vi "Enqueue Message.vi"   [LabVIEW 2024, in "AA PM Message Queue.lvlib"]
doc: "For a regular message, enqueue the message. For a priority message, enqueue it at the front of the queue."
uses:
  AA PM Message Queue.lvlib
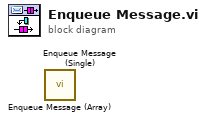
[diagram p0: block diagram]
diagram:
  n1 = call "Enqueue Message (Array).vi"() -> ()  [unwired: 10 in, 2 out]
  n2 = call "Enqueue Message (Single).vi"() -> ()  [unwired: 10 in, 2 out]
